vi "XML_FF_writeHeader.vi"(8 "error in (no error)":errorcluster, 10 "XML_FF_Header":T1, 11 "DOM document in":refnum<k20>) -> (0 "error out":errorcluster, 3 "DOM document out":refnum<k20>)   [LabVIEW 2016, in "XML_EEG_Features.lvlib"]
uses:
  XML_EEG_Features.lvlib
  XML_FF_Header.ctl
  <resource>/objmgr/DOMUserDefRef.rc
  <vilib>/xml/NI_XML.lvlib
panel:
  # "This VI is a part of BCI Design library, http://www.ru-bci.org \nCopyright © 2020, Sotnikov Peter, All rights reserved. License: GNU GPLv3"
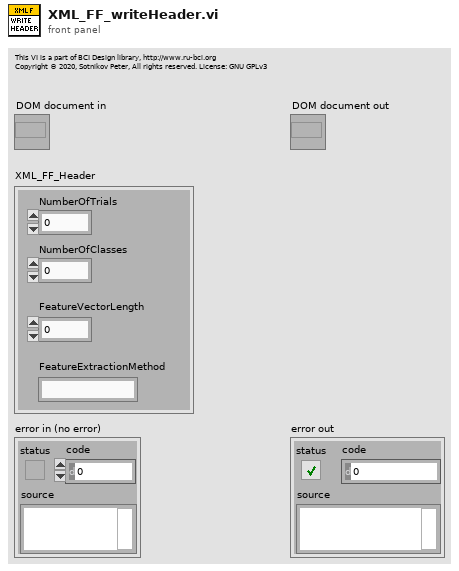
[diagram p1: front panel]
types:
  T1 = typedef "XML_EEG_Features.lvlib/XML_FF_Header.ctl" = cluster{"NumberOfTrials":i32, "NumberOfClasses":i32, "FeatureVectorLength":i32, "FeatureExtractionMethod":string}
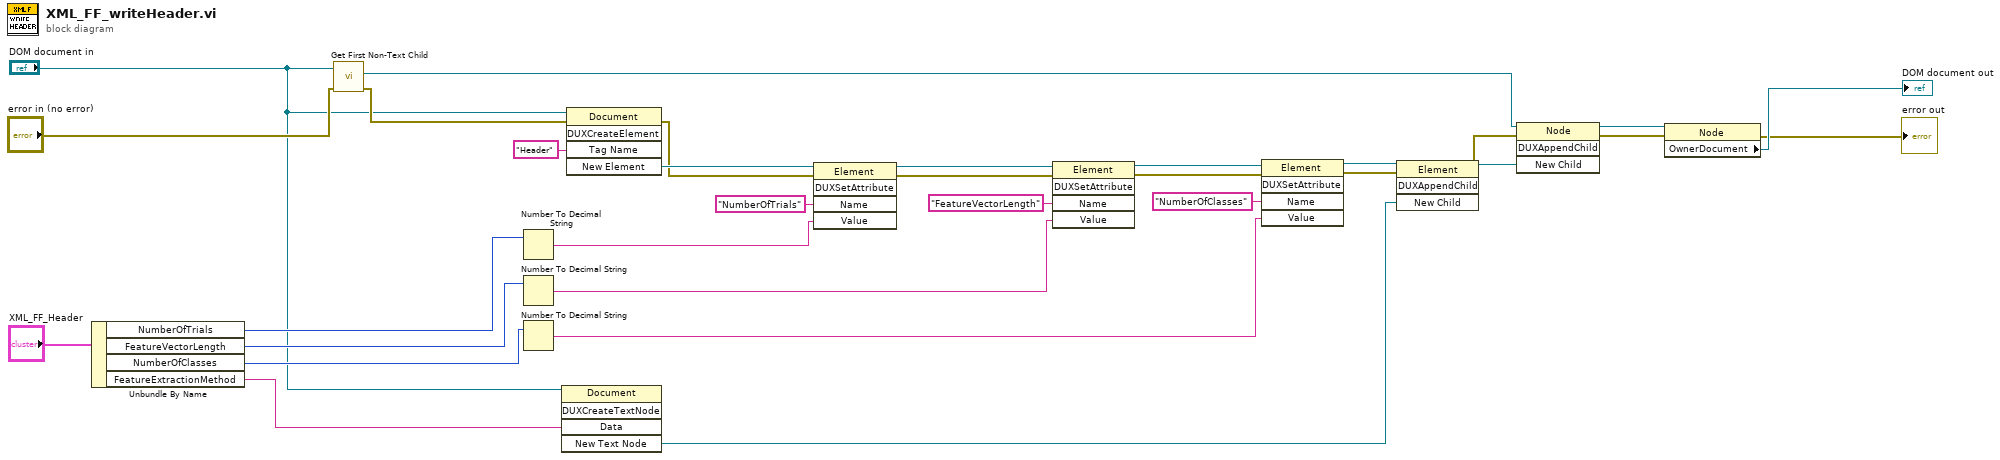
[diagram p0: block diagram]
diagram:
  n1 = Unbundle By Name("XML_FF_Header") -> ("NumberOfTrials"=w27:i32, "FeatureVectorLength"=w21:i32, "NumberOfClasses"=w10:i32, "FeatureExtractionMethod"=w16:string)
  n2 = call <vilib>:"Get First Non-Text Child.vi"("error in (no error)"="error in (no error)", "node in"="DOM document in") -> ("error out"=w7:errorcluster, "child node"=w6:refnum<k20>)  [unwired: 6 in, 2 out]
  n3 = Number To Decimal String(number=w27) -> (decimal integer string=w26:string)  [unwired: 1 in]
  n4 = Number To Decimal String(number=w21) -> (decimal integer string=w20:string)  [unwired: 1 in]
  n5 = Number To Decimal String(number=w10) -> (decimal integer string=w9:string)  [unwired: 1 in]
  n6 = invoke class="Document" method="DUXCreateTextNode"(reference="DOM document in", "Data"=w16) -> ("New Text Node"=w19:refnum<k20>)  [unwired: 3 in, 4 out]
  n7 = invoke class="Document" method="DUXCreateElement"(reference="DOM document in", error in=w7, "Tag Name"="Header") -> (error out=w24:errorcluster, "New Element"=w30:refnum<k20>)  [unwired: 2 in, 3 out]
  n8 = invoke class="Element" method="DUXSetAttribute"(reference=w30, error in=w24, "Name"="NumberOfTrials", "Value"=w26) -> (reference out=w25:refnum<k20>, error out=w23:errorcluster)  [unwired: 1 in, 3 out]
  n9 = invoke class="Element" method="DUXSetAttribute"(reference=w25, error in=w23, "Name"="FeatureVectorLength", "Value"=w20) -> (reference out=w15:refnum<k20>, error out=w14:errorcluster)  [unwired: 1 in, 3 out]
  n10 = invoke class="Element" method="DUXSetAttribute"(reference=w15, error in=w14, "Name"="NumberOfClasses", "Value"=w9) -> (reference out=w12:refnum<k20>, error out=w13:errorcluster)  [unwired: 1 in, 3 out]
  n11 = invoke class="Element" method="DUXAppendChild"(reference=w12, error in=w13, "New Child"=w19) -> (reference out=w18:refnum<k20>, error out=w17:errorcluster)  [unwired: 1 in, 2 out]
  n12 = invoke class="Node" method="DUXAppendChild"(reference=w6, error in=w17, "New Child"=w18) -> (reference out=w4:refnum<k20>, error out=w3:errorcluster)  [unwired: 1 in, 2 out]
  n13 = property class="Node"(reference=w4, error in=w3) -> (error out=→"error out":errorcluster, "OwnerDocument"=→"DOM document out":refnum<k20>)  [unwired: 1 out]
